vi "Set Config Digitals (Batch).vi"(0 "connection ID":refnum<k16>, 1 "address":u32, 2 "port":u16, 5 "Mask":bool[](array[boolean])=[TRUE, TRUE, TRUE, TRUE, TRUE, TRUE, TRUE, TRUE, TRUE, TRUE, TRUE, TRUE, TRUE, TRUE, TRUE, TRUE], 7 "Digital Mode":T1=73 items=["Output"=79, "Input_Pullup"=80, "Input"=73], 9 "timeout ms (1000)":i32=1000, 11 "error in (no error)":errorcluster) -> (4 "connection ID out":refnum<k16>, 6 "received data":string, 15 "error out":errorcluster)   [LabVIEW 2016, in "instr.lvlib"]
doc: "Sets all digital io to given digital mode. Batch operation."
uses:
  instr.lvlib
  Digital Mode.ctl
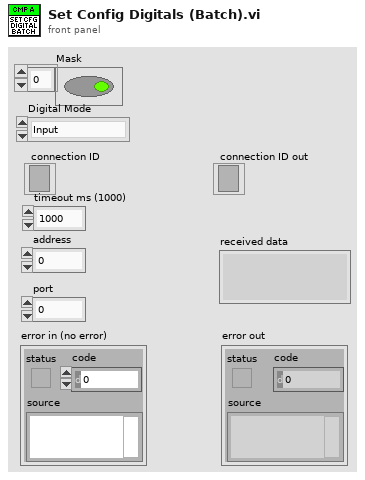
[diagram p1: front panel]
types:
  T1 = typedef "instr.lvlib/Digital Mode.ctl" = u16
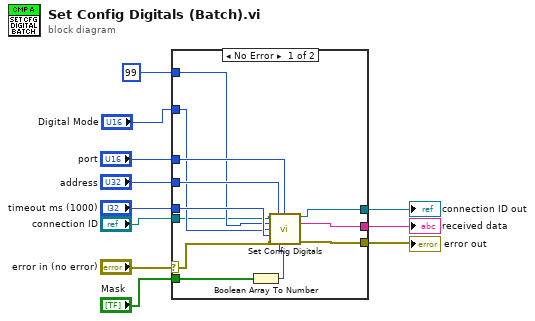
[diagram p0: block diagram]
diagram:
  n1 = case shown="No Error" "error in (no error)" {
    selector: "error in (no error)" -> [w19 w25]
    tunnel: [w22 w25] -> w11
    tunnel: [w21 _] -> w9
    tunnel: "timeout ms (1000)" -> [w17 _]
    tunnel: "connection ID" -> [w12 w24]
    tunnel: [w20 w24] -> w6
    tunnel: u16 99 ("Digital Number") -> [w13 _]
    tunnel: "Digital Mode" -> [w14 _]
    tunnel: "address" -> [w16 _]
    tunnel: "port" -> [w15 _]
    tunnel: "Mask" -> [w23 _]
    frame No Error {
      n2 = Boolean Array To Number(Boolean array=w23) -> (number=w18:u32)
      n3 = call "Set Config Digitals.vi"("connection ID"=w12, "address"=w16, "port"=w15, "Digital Number"=w13, "Digital Mode"=w14, "timeout ms (1000)"=w17, "error in (no error)"=w19, "mask"=w18) -> ("connection ID out"=w20:refnum<k16>, "received data"=w21:string, "error out"=w22:errorcluster)  [unwired: 5 in]
    }
    frame Error {
    }
  }
  "error out" <- w11
  "received data" <- w9
  "connection ID out" <- w6
